vi "Process.vi"(8 "error in":errorcluster, 11 "Logger.Error":refnum<class "Logger.Error.lvclass">) -> (0 "error out":errorcluster, 3 "Logger.Error out":refnum<class "Logger.Error.lvclass">)   [LabVIEW 2019, in "Logger.Error.lvclass"]
doc: "---------------------------------------------------------------\nJKI State Machine Objects™\nhttp://jki.net/state-machine-objects/\nCopyright (C) 2005-2015, JKI <info@jki.net>\nALL RIGHTS RESERVED"
uses:
  Logger.Error.lvclass
  C:/Program Files (x86)/National Instruments/LabVIEW 2019/vi.lib/JKI/JKI SMO/SMO/SMO.lvclass
  C:/Users/patrick/Documents/GitHub/Instrument-Framework/lvsrc/SMOs/Logger/Logger.lvclass
  <vilib>/JKI/JKI SMO/SMO/SMO.lvclass
  <vilib>/JKI/JKI SMO/SMO/SMO.lvclass/SMO.ctl
  Logger.Error.lvclass/Logger.Error.ctl
  <vilib>/JKI/JKI SMO/SMO/Private/ReftoDVR--SMO.vi
  <vilib>/Utility/file.llb/Write Delimited Spreadsheet (string).vi
  <userlib>/LevyLab/Logger/Logger.lvclass
panel:
  out "Status":string
  out "State History":string
  # "error Logger"
  # "For instructions on how to use the JKI State Machine Objects, examples and video tutorials, visit:\nhttp://jki.net/state-machine-objects/\n\nJKI State Machine Objects™\nhttp://jki.net/state-machine-objects/\nCopyright (C) 2005-2015, JKI <info@jki.net>\nALL RIGHTS RESERVED"
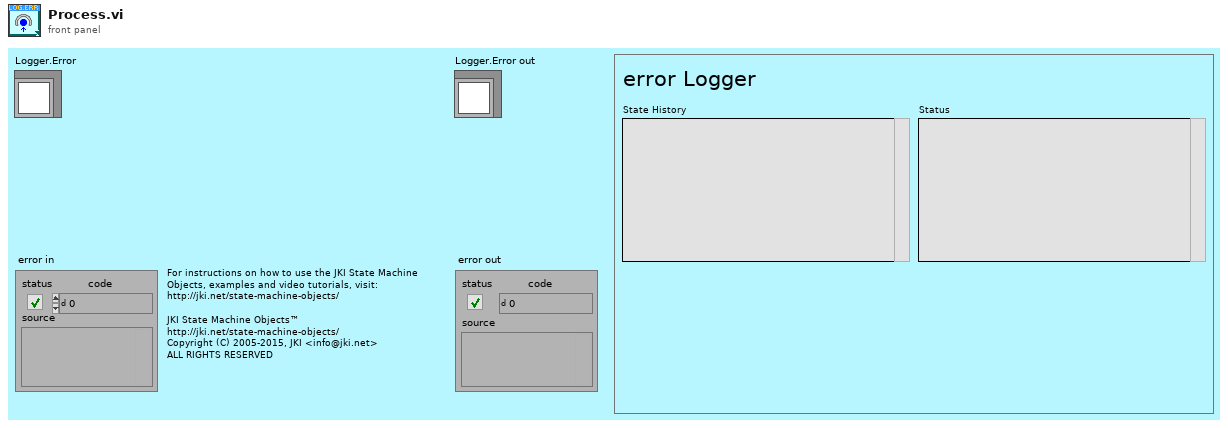
[diagram p1: front panel]
types:
  T1 = enum32{"invalid app kind", "Development System", "Run Time System", "Student Edition", "Embedded LabVIEW", "Evaluation", "Custom"}
  T2 = enum32{"Invalid", "Standard", "Closed", "Hidden", "Minimized", "Maximized"}
  T3 = cluster{"Core":cluster{"Current VI Reference":refnum<vi>, "Close Panel on Exit?":bool, "Last Error":cluster{"error":errorcluster, "previous state":string, "remaining states":string}, "Shutdown?":bool}, "SelfRef":refnum<class "Logger.Error.lvclass">, "path":path, "Debug Mode?":bool, "SMOs":refnum<class "SMO.lvclass">[], "error to log":errorcluster}
  T4 = cluster{"Current VI Reference":refnum<vi>, "Close Panel on Exit?":bool, "Last Error":cluster{"error":errorcluster, "previous state":string, "remaining states":string}, "Shutdown?":bool}
  T5 = typedef "SMO.lvclass/Protected Events.ctl" = cluster{"StopProcesses":refnum<user-event>, "AbortProcesses":refnum<user-event>, "Config Changed":refnum<user-event>, "Dependency":refnum<user-event>}
  T6 = typedef "SMO.lvclass/Public Events.ctl" = cluster{"Error":refnum<user-event>, "State":refnum<user-event>, "Reserve State":refnum<user-event>}
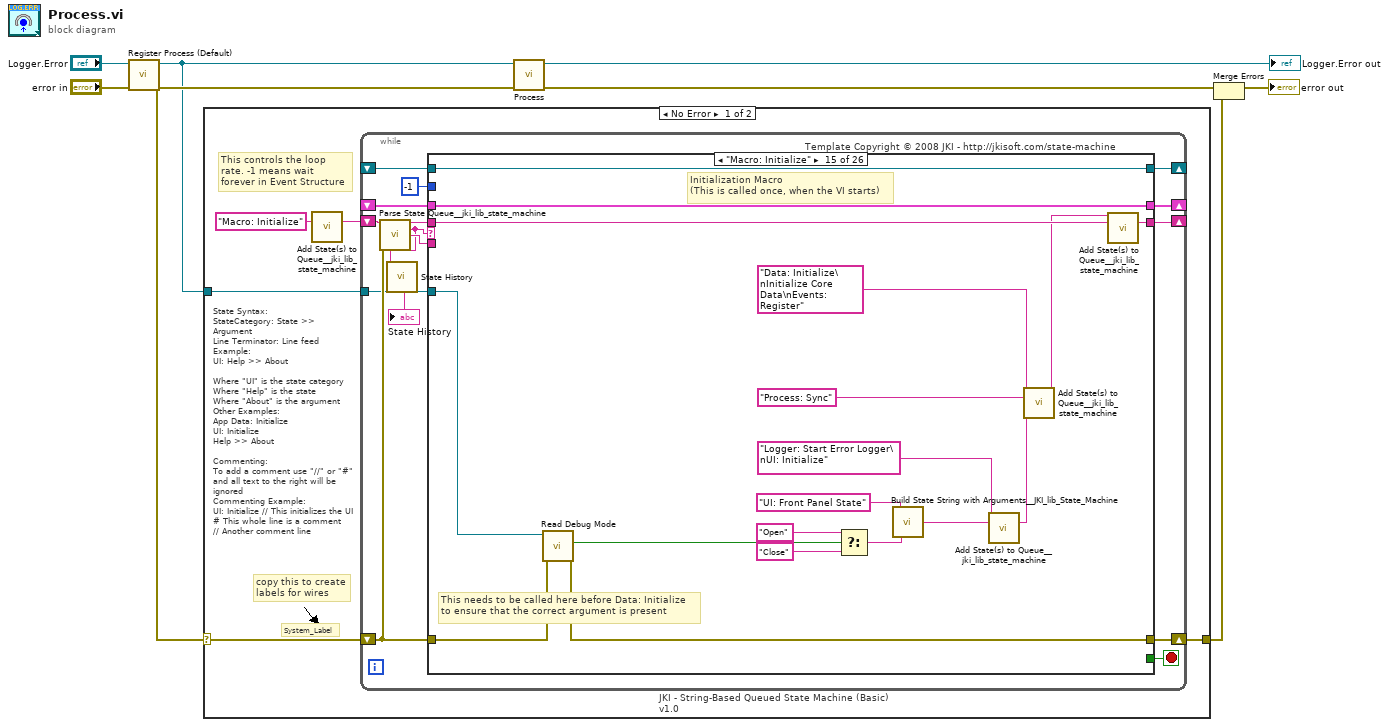
[diagram p0: block diagram]
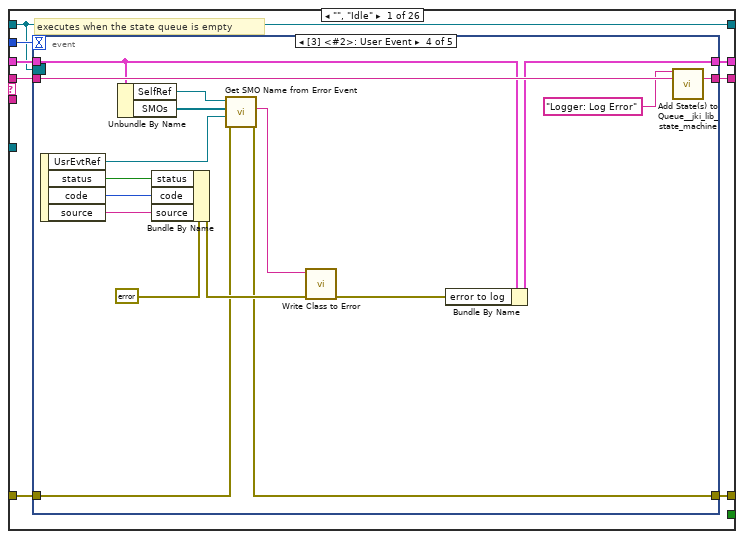
[diagram p2: hidden frame]
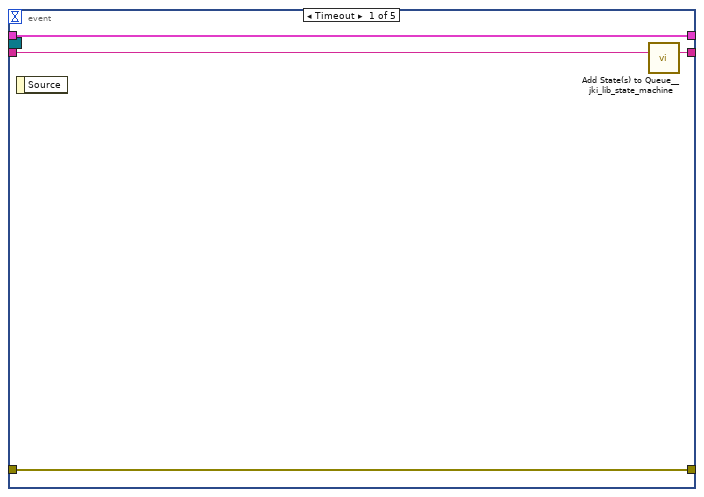
[diagram p3: hidden frame]
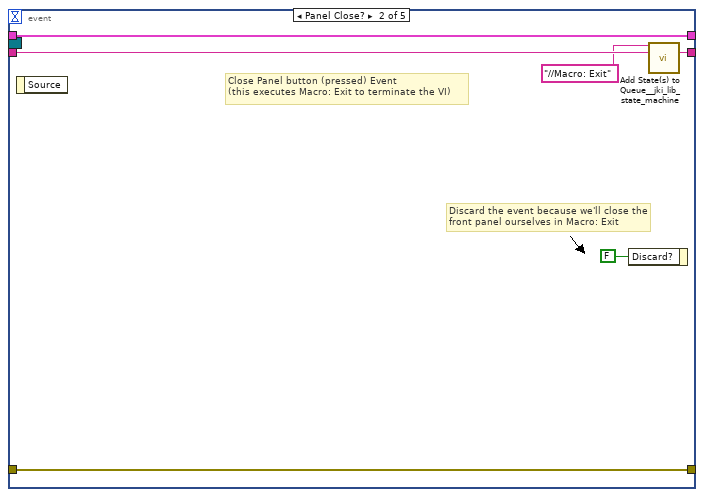
[diagram p4: hidden frame]
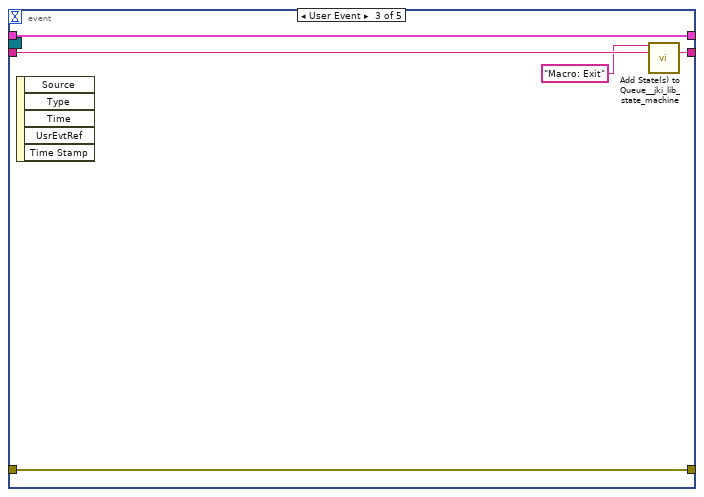
[diagram p5: hidden frame]
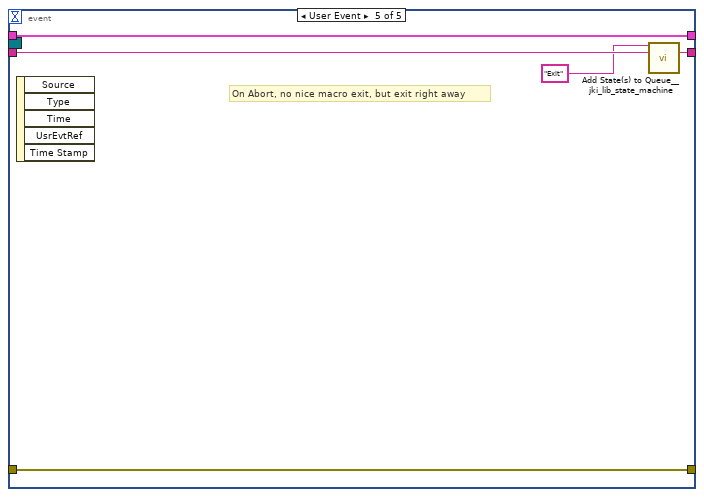
[diagram p6: hidden frame]
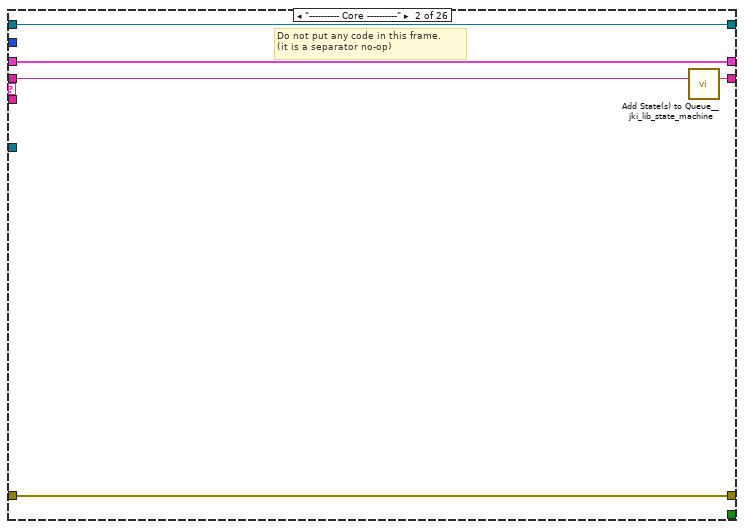
[diagram p7: hidden frame]
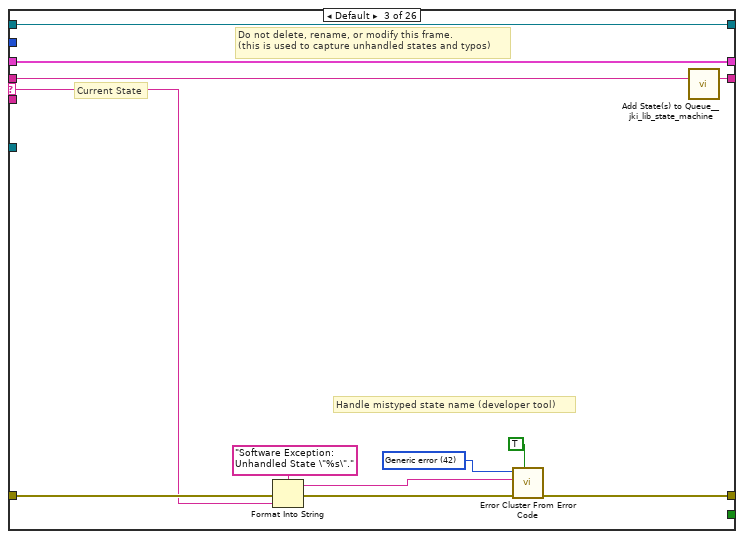
[diagram p8: hidden frame]
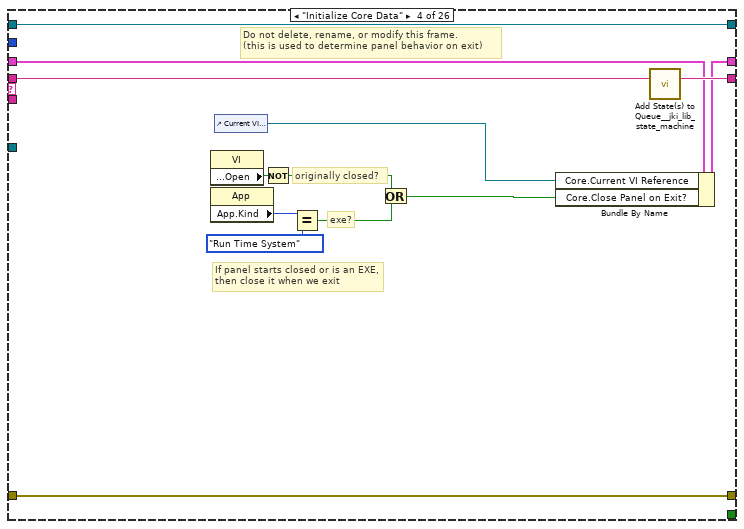
[diagram p9: hidden frame]
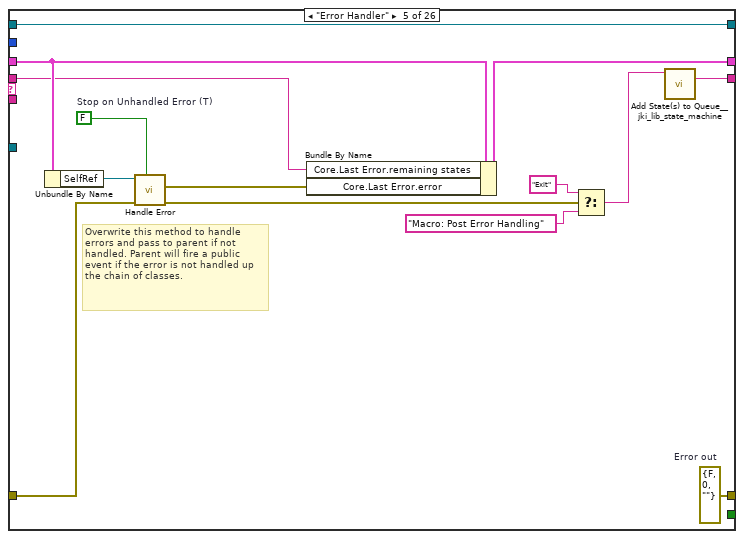
[diagram p10: hidden frame]
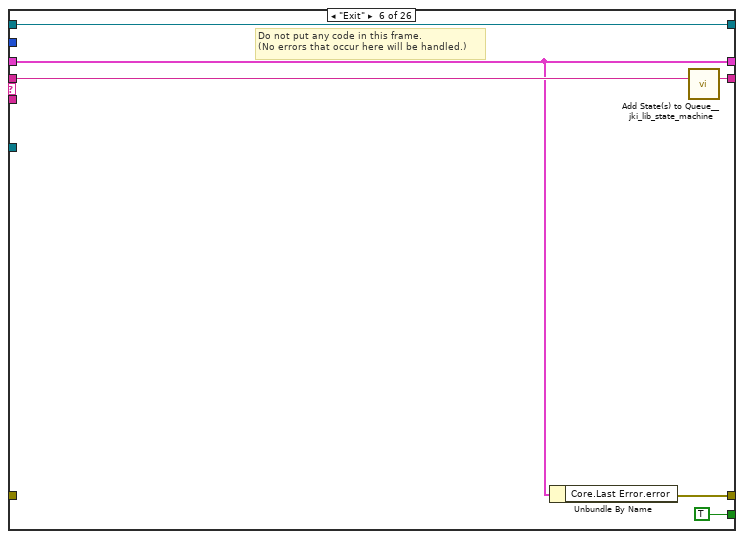
[diagram p11: hidden frame]
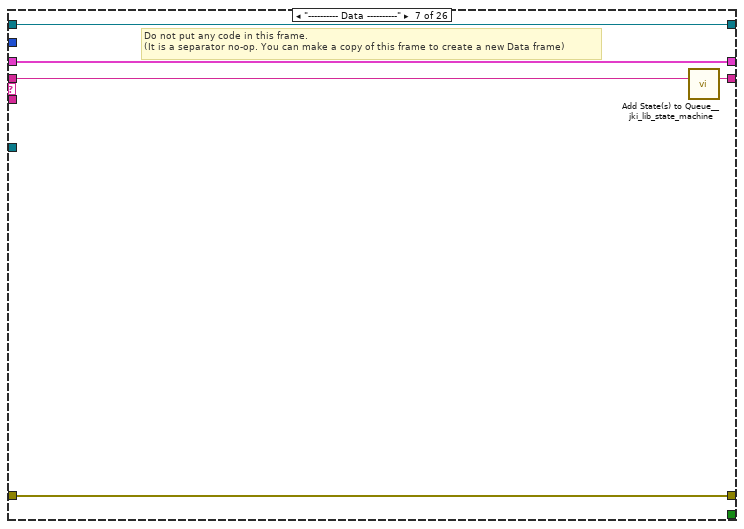
[diagram p12: hidden frame]
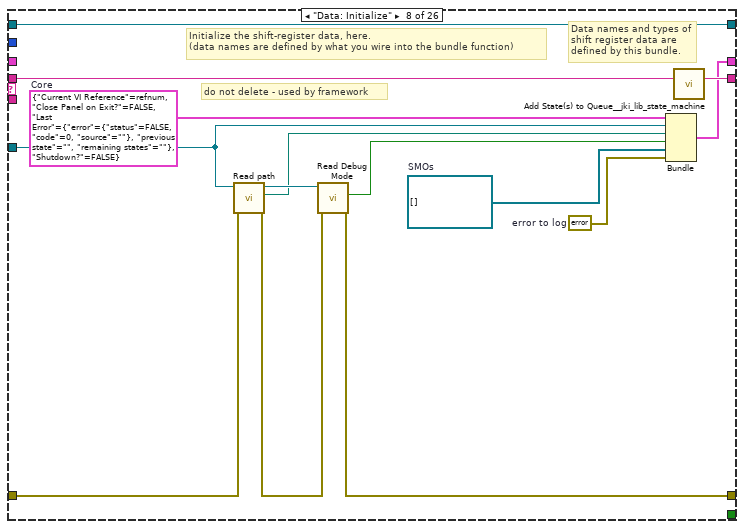
[diagram p13: hidden frame]
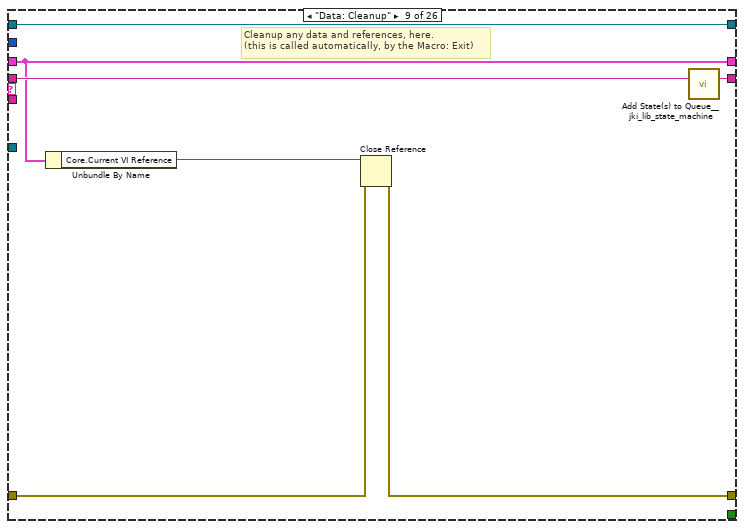
[diagram p14: hidden frame]
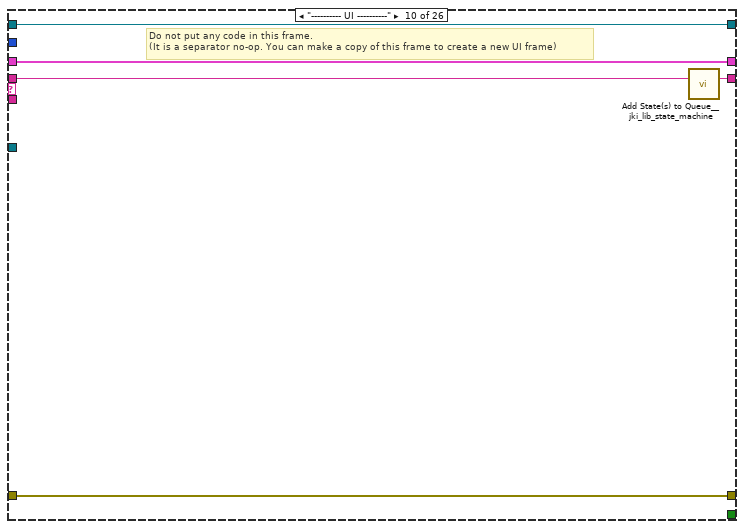
[diagram p15: hidden frame]
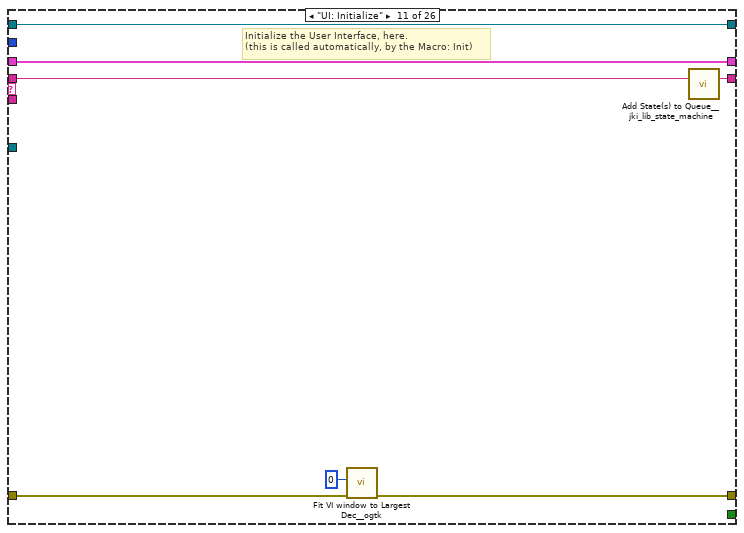
[diagram p16: hidden frame]
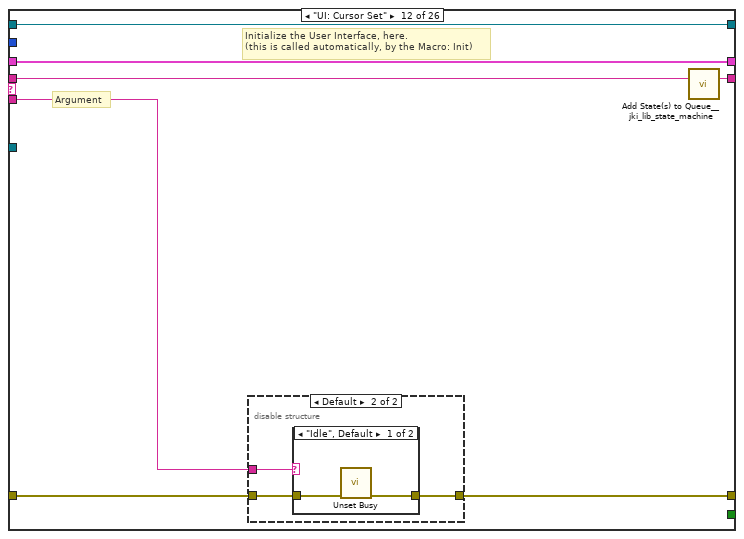
[diagram p17: hidden frame]
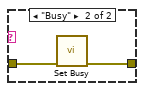
[diagram p19: hidden frame]
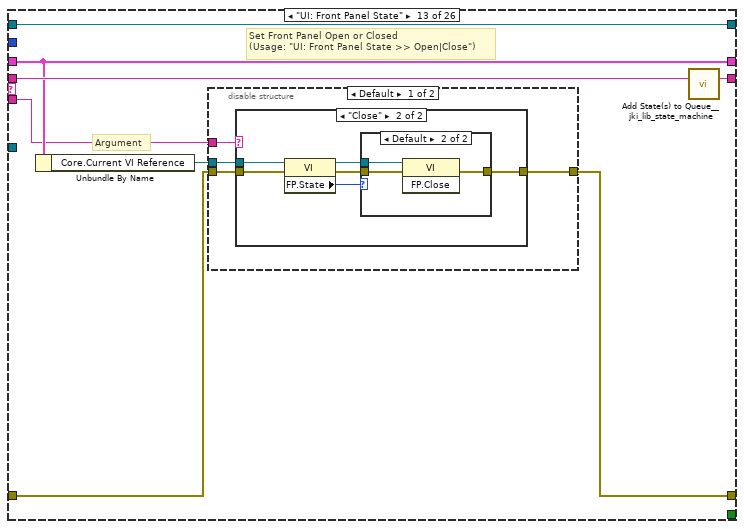
[diagram p20: hidden frame]
diagram:
  n1 = call <vilib>:"Register Process (Default).vi"("error in (no error)"="error in", "SMO"="Logger.Error") -> ("error out"=w5:errorcluster, "SelfRef"=w4:refnum<class "Logger.Error.lvclass">)  [unwired: 8 in]
  n2 = case shown="No Error" w5 {
    selector: w5 -> [w10 w358]
    tunnel: w4 -> [w11 _]
    tunnel: [w9 w358] -> w1
    frame No Error {
      # "State Syntax:\nStateCategory: State >> Argument\nLine Terminator: Line feed\nExample:\nUI: Help >> About\n\nWhere \"UI\" is the state category\nWhere \"Help\" is the state\nWhere \"About\" is the argument\nOther Examples:\nApp Data: Initialize\nUI: Initialize\nHelp >> About\n\nCommenting:\nTo add a comment use \"//\" or \"#\" and all text to the right will be ignored\nCommenting Example:\nUI: Initialize // This initializes the UI\n# This whole line is a comment\n// Another comment line"
      # "copy this to create labels for wires"
      # "This controls the loop rate. -1 means wait forever in Event Structure"
      # "System_Label"
      n3 = call <vilib>:"Add State(s) to Queue__jki_lib_state_machine.vi"("State(s) in (\"\")"="Macro: Initialize") -> ("States Out"=w13:string)  [unwired: 14 in]
      n4 = while "JKI - String-Based Queued State Machine (Basic) v1.0" {
        shift-right: [w22] -> _
        shift-left: _ -> [w14]
        shift-right: [w25] -> w9
        shift-left: w10 -> [w20]
        shift-right: [w24] -> _
        shift-left: w13 -> [w26]
        tunnel: w11 -> [w19]
        shift-right: [w18] -> _
        shift-left: _ -> [w17]
        stop <- w23 stop-if-true
        # "Template Copyright © 2008 JKI - http://jkisoft.com/state-machine"
        n5 = call <vilib>:"Parse State Queue__jki_lib_state_machine.vi"("State Queue"=w26, "Error In (no error)"=w20) -> ("Remaining States"=w28:string, "Current State"=w15:string, "Arguments"=w27:string)  [unwired: 11 in]
        n6 = call <userlib>:"State History.vi"("Current State"=w15) -> ("History"=→"State History":string)  [unwired: 10 in]
        n7 = case shown="\"Macro: Initialize\"" w15 {
          selector: w15 -> [_ _ w80 _ _ _ _ _ _ _ _ _ _ _ _ _ _ _ _ _ _ _ _ _ _ _]
          tunnel: w28 -> [w36 w78 w84 w103 w106 w123 w128 w142 w149 w154 w161 w168 w184 w216 w234 w246 w270 w275 w286 w291 w308 w319 w324 w333 w340 w357]
          tunnel: w27 -> [_ _ _ _ _ _ _ _ _ _ _ w162 w178 _ _ _ _ _ _ _ _ _ _ _ _ _]
          tunnel: [w33 w76 w86 w100 w113 w118 w126 w133 w145 w152 w156 w163 w181 w214 w219 w244 w268 w273 w277 w289 w304 w315 w320 w329 w334 w342] -> w25
          tunnel: w20 -> [w32 w76 w85 w100 w114 _ w126 w129 w146 w152 w155 w164 w182 w214 w218 w244 w268 w273 w278 w289 w295 w315 w320 w330 w335 w347]
          tunnel: [w35 w77 w83 w102 w117 w122 w127 w141 w148 w153 w160 w167 w183 w215 w233 w245 w269 w274 w285 w290 w307 w318 w323 w332 w339 w356] -> w24
          tunnel: [_ _ _ _ _ TRUE _ _ _ _ _ _ _ _ _ _ _ _ _ _ _ _ _ _ _ _] -> w23
          tunnel: [w31 w75 w82 w101 w111 w119 w125 w140 w144 w151 w159 w166 w180 w213 w222 w236 w262 w272 w283 w288 w298 w317 w322 w326 w337 w354] -> w22
          tunnel: -1 ("Timeout") -> [w30 _ _ _ _ _ _ _ _ _ _ _ _ _ _ _ _ _ _ _ _ _ _ _ _ _]
          tunnel: w19 -> [_ _ _ _ _ _ _ w130 _ _ _ _ _ _ w220 _ _ _ _ _ _ _ _ _ _ _]
          tunnel: [w29 w74 w79 w91 w116 w120 w124 w139 w143 w150 w158 w165 w177 w212 w232 w243 w263 w271 w284 w287 w306 w316 w321 w331 w338 w355] -> w18
          tunnel: w17 -> [w29 w74 w79 w91 w116 w120 w124 w139 w143 w150 w158 w165 w177 w212 w232 w243 w263 w271 w284 w287 _ w316 w321 w331 w338 w355]
          tunnel: w14 -> [w34 w75 w82 w94 w112 w119 w125 _ w144 w151 w159 w166 w180 w213 w222 w235 w262 w272 w283 w288 w299 w317 w322 w325 w337 w354]
          frame "", "Idle" {
            # "executes when the state queue is empty"
            n8 = event shown="[3] <#2>: User Event" {
              selector: w29 -> [_ _ _ _ _]
              dyn-events: _ -> [_ _ _ _ _]
              timeout: w30 -> [_ _ _ _ _]
              tunnel: w36 -> [w40 w46 w51 w68 w73]
              tunnel: [w39 w45 w50 w67 w72] -> w35
              tunnel: w34 -> [w38 w43 w48 w55 w70]
              tunnel: [w37 w44 w49 w57 w71] -> w33
              tunnel: w32 -> [w37 w44 w49 w58 w71]
              tunnel: [w38 w43 w48 w56 w70] -> w31
              event Timeout {
                n9 = event-data() -> ()  [unwired: 1 in, 1 out]
                n10 = call <vilib>:"Add State(s) to Queue__jki_lib_state_machine.vi"("State(s) in (\"\")"=w40) -> ("States Out"=w39:string)  [unwired: 14 in]
              }
              event Panel Close? {
                # "Discard the event because we'll close the front panel ourselves in Macro: Exit"
                # "Close Panel button (pressed) Event\n(this executes Macro: Exit to terminate the VI)"
                n11 = event-data() -> ()  [unwired: 1 in, 1 out]
                n12 = event-data("Discard?"=FALSE) -> ()  [unwired: 1 in, 1 out]
                n13 = call <vilib>:"Add State(s) to Queue__jki_lib_state_machine.vi"("State(s) in Front (\"\")"="//Macro: Exit", "State(s) in (\"\")"=w46) -> ("States Out"=w45:string)  [unwired: 13 in]
              }
              event User Event {
                n14 = event-data() -> ()  [unwired: 1 in, 5 out]
                n15 = call <vilib>:"Add State(s) to Queue__jki_lib_state_machine.vi"("State(s) in Front (\"\")"="Macro: Exit", "State(s) in (\"\")"=w51) -> ("States Out"=w50:string)  [unwired: 13 in]
              }
              event User Event {
                n16 = event-data() -> ("UsrEvtRef"=w62:refnum<user-event>, "status"=w66:bool, "code"=w65:i32, "source"=w64:string)  [unwired: 1 in]
                n17 = Unbundle By Name(w55) -> ("SelfRef"=w52:refnum<class "Logger.Error.lvclass">, "SMOs"=w63:refnum<class "SMO.lvclass">[])
                n18 = Bundle By Name(cluster=errorcluster {"status"=FALSE, "code"=0, "source"=""} ("error in (no error)"), "status"=w66, "code"=w65, "source"=w64) -> (w60:errorcluster)
                n19 = call "Get SMO Name from Error Event.vi"("error in (no error)"=w58, "Error"=w62, "SMOs"=w63, "Logger.Error"=w52) -> ("error out"=w57:errorcluster, "class:SMO name"=w61:string)  [unwired: 5 in, 1 out]
                n20 = call "Write Class to Error.vi"("Error in"=w60, "Calling Class"=w61) -> ("Error out"=w54:errorcluster)  [unwired: 9 in]
                n21 = Bundle By Name(cluster=w55, "error to log"=w54) -> (w56:T3)
                n22 = call <vilib>:"Add State(s) to Queue__jki_lib_state_machine.vi"("State(s) in Front (\"\")"="Logger: Log Error" ("State(s) in Front (\"\")"), "State(s) in (\"\")"=w68) -> ("States Out"=w67:string)  [unwired: 13 in]
              }
              event User Event {
                # "On Abort, no nice macro exit, but exit right away"
                n23 = event-data() -> ()  [unwired: 1 in, 5 out]
                n24 = call <vilib>:"Add State(s) to Queue__jki_lib_state_machine.vi"("State(s) in Front (\"\")"="Exit", "State(s) in (\"\")"=w73) -> ("States Out"=w72:string)  [unwired: 13 in]
              }
            }
          }
          frame "---------- Core ----------" {
            # "Do not put any code in this frame.\n(it is a separator no-op)"
            n25 = call <vilib>:"Add State(s) to Queue__jki_lib_state_machine.vi"("State(s) in (\"\")"=w78) -> ("States Out"=w77:string)  [unwired: 14 in]
          }
          frame Default {
            w89 = 42 items=["No error", "Argument error", "Memory is full", "Out of zone", "End of file", "File already open", "Generic file I/O error", "File not found", "File permission error", "Disk is full", "Duplicate path", "Too many files open", "System feature not enabled", "Resource file not found", "Cannot add resource", "Resource not found", "Image not found", "Image memory error", "Pen does not exist", "Config type invalid", "Config token not found", "Config parse error", "Config memory error", "Bad external code format", "Bad external code offset", "External code not present", "Null window", "Destroy window error", "Null menu", "Print aborted", "Bad print record", "Print driver error", "Windows error during printing", "Memory error during printing", "Print dialog error", "Generic print error", "Invalid device refnum", "Device not found", "Device parameter error", "Device unit error", "Cannot open device", "Device call aborted", "Generic error", "Cancelled by user", "Object ID too low", "Object ID too high", "Object not in heap", "Unknown heap", "Unknown object (invalid DefProc)", "Unknown object (DefProc not in table)", "Message out of range", "Invalid (null) method", "Unknown message", "Manager call not supported", "Bad address", "Network operation in progress", "Network operation timed out", "Connection is busy", "Network attribute not supported", "Network error", "Address in use", "System out of memory", "Connection aborted", "Connection refused", "Not connected", "Already connected", "Connection closed", "Initialization error (interapplication manager)", "Bad occurrence", "Wait on unbound occurrence handler", "Occurrence queue overflow", "Datalog type conflict", "Unused", "Unrecognized type (interapplication manager)", "Memory corrupt", "Failed to make temporary DLL", "Old CIN version", "Drag socket not found", "Failed to load drop-object", "Failed to register OLE object", "Failed to release OLE object", "Format specifier type mismatch", "Unknown format specifier", "Too few format specifiers", "Too many format specifiers", "Scan failed", "Newer CIN version", "Error converting to variant", "Runtime menu error", "Password tampered", "Variant attribute not found", "Incompatible variant data type", "Event data is not available", "Event Store is not present", "Occurrence is not found", "Event Queue is not created", "Event info is not available", "Refnum passed is NULL", "Error retrieving Class GUID", "Error retrieving CoClass GUID", "Error retrieving TypeLib GUID.", "Bad built application magic bytes.", "Specific driver is different from the specific driver associated with the Logical Name.", "There is no session opened to the class driver.", "Max Error", "MAX - Error with config objects", "MAX - Error loading configuration", "MAX - Group not supported"]
            # "Current State"
            # "Do not delete, rename, or modify this frame.\n(this is used to capture unhandled states and typos)"
            # "Handle mistyped state name (developer tool)"
            n26 = Format Into String(format string="Software Exception: Unhandled State \"%s\"." ("message"), error in=w85, w80) -> (resulting string=w88:string, error out=w87:errorcluster)  [unwired: 1 in]
            n27 = call <vilib>:"Error Cluster From Error Code.vi"("show call chain? (False)"=TRUE, "error in (no error)"=w87, "error message (\"\")"=w88, "error code (0)"=w89) -> ("error out"=w86:errorcluster)  [unwired: 5 in]
            n28 = call <vilib>:"Add State(s) to Queue__jki_lib_state_machine.vi"("State(s) in (\"\")"=w84) -> ("States Out"=w83:string)  [unwired: 14 in]
          }
          frame "Initialize Core Data" {
            # "Do not delete, rename, or modify this frame.\n(this is used to determine panel behavior on exit)"
            # "originally closed?"
            # "exe?"
            # "If panel starts closed or is an EXE, then close it when we exit"
            n29 = property class="VI"() -> ("Front Panel.Open"=w99:bool)  [unwired: 2 in, 2 out]
            n30 = property class="App"() -> ("App.Kind"=w98:T1)  [unwired: 2 in, 2 out]
            n31 = control-ref of="Current VI Reference"() -> (w92:refnum<vi>)
            n32 = Not(x=w99) -> (.not. x?=w96:bool)
            n33 = Equal?(x=w98, y=T1."Run Time System" ("Application:Kind")) -> (x = y?=w95:bool)
            n34 = Or(x=w96, y=w95) -> (x .or. y?=w93:bool)
            n35 = Bundle By Name(cluster=w94, "Core.Current VI Reference"=w92, "Core.Close Panel on Exit?"=w93) -> (w101:T3)
            n36 = call <vilib>:"Add State(s) to Queue__jki_lib_state_machine.vi"("State(s) in (\"\")"=w103) -> ("States Out"=w102:string)  [unwired: 14 in]
          }
          frame "Error Handler" {
            w107 = FALSE  # Stop on Unhandled Error (T)
            w113 = errorcluster {"status"=FALSE, "code"=0, "source"=""}  # Error out
            # "Overwrite this method to handle errors and pass to parent if not handled. Parent will fire a public event if the error is not handled up the chain of classes."
            n37 = Unbundle By Name(w112) -> ("SelfRef"=w115:refnum<class "Logger.Error.lvclass">)
            n38 = call-dynamic "Handle Error.vi"("Stop on Unhandled Error (T)"=w107, "error in"=w114, "SMO"=w115) -> ("handling error"=w108:errorcluster, "Unhandled error"=w104:errorcluster)  [unwired: 6 in, 1 out]
            n39 = Bundle By Name(cluster=w112, "Core.Last Error.remaining states"=w106, "Core.Last Error.error"=w104) -> (w111:T3)
            n40 = Select(t="Exit", s=w108, f="Macro: Post Error Handling") -> (s? t:f=w110:string)
            n41 = call <vilib>:"Add State(s) to Queue__jki_lib_state_machine.vi"("State(s) in Front (\"\")"=w110) -> ("States Out"=w117:string)  [unwired: 14 in]
          }
          frame "Exit" {
            # "Do not put any code in this frame.\n(No errors that occur here will be handled.)"
            n42 = Unbundle By Name(w119) -> ("Core.Last Error.error"=w118:errorcluster)
            n43 = call <vilib>:"Add State(s) to Queue__jki_lib_state_machine.vi"("State(s) in (\"\")"=w123) -> ("States Out"=w122:string)  [unwired: 14 in]
          }
          frame "---------- Data ----------" {
            # "Do not put any code in this frame.\n(It is a separator no-op. You can make a copy of this frame to create a new Data frame)"
            n44 = call <vilib>:"Add State(s) to Queue__jki_lib_state_machine.vi"("State(s) in (\"\")"=w128) -> ("States Out"=w127:string)  [unwired: 14 in]
          }
          frame "Data: Initialize" {
            w131 = errorcluster {"status"=FALSE, "code"=0, "source"=""}  # error to log
            w132 = refnum<class "SMO.lvclass">[] []  # SMOs
            w138 = T4 {"Current VI Reference"=refnum, "Close Panel on Exit?"=FALSE, "Last Error"={"error"={"status"=FALSE, "code"=0, "source"=""}, "previous state"="", "remaining states"=""}, "Shutdown?"=FALSE}  # Core
            # "do not delete - used by framework"
            # "Data names and types of shift register data are defined by this bundle."
            # "Initialize the shift-register data, here.\n(data names are defined by what you wire into the bundle function)"
            n45 = call-dynamic "Read path.vi"("error in (no error)"=w129, "Logger in"=w130) -> ("error out"=w135:errorcluster, "path"=w134:path, "Logger out"=w137:refnum<class "Logger.Error.lvclass">)  [unwired: 7 in]
            n46 = call <userlib>:"Read Debug Mode.vi"("error in (no error)"=w135, "Logger in"=w137) -> ("error out"=w133:errorcluster, "Debug Mode?"=w136:bool)  [unwired: 7 in, 1 out]
            n47 = Bundle("Core"=w138, "SelfRef"=w130, "path"=w134, "Debug Mode?"=w136, "SMOs"=w132, "error to log"=w131) -> (w140:T3)  [unwired: 1 in]
            n48 = call <vilib>:"Add State(s) to Queue__jki_lib_state_machine.vi"("State(s) in (\"\")"=w142) -> ("States Out"=w141:string)  [unwired: 14 in]
          }
          frame "Data: Cleanup" {
            # "Cleanup any data and references, here.\n(this is called automatically, by the Macro: Exit)"
            n49 = Unbundle By Name(w144) -> ("Core.Current VI Reference"=w147:refnum<vi>)
            n50 = Close Reference(reference=w147, error in (no error)=w146) -> (error out=w145:errorcluster)
            n51 = call <vilib>:"Add State(s) to Queue__jki_lib_state_machine.vi"("State(s) in (\"\")"=w149) -> ("States Out"=w148:string)  [unwired: 14 in]
          }
          frame "---------- UI ----------" {
            # "Do not put any code in this frame.\n(It is a separator no-op. You can make a copy of this frame to create a new UI frame)"
            n52 = call <vilib>:"Add State(s) to Queue__jki_lib_state_machine.vi"("State(s) in (\"\")"=w154) -> ("States Out"=w153:string)  [unwired: 14 in]
          }
          frame "UI: Initialize" {
            # "Initialize the User Interface, here.\n(this is called automatically, by the Macro: Init)"
            n53 = call <userlib>:"Fit VI window to Largest Dec__ogtk.vi"("error in (no error)"=w155, "border spacing (2 px)"=0) -> ("error out"=w156:errorcluster)  [unwired: 4 in, 1 out]
            n54 = call <vilib>:"Add State(s) to Queue__jki_lib_state_machine.vi"("State(s) in (\"\")"=w161) -> ("States Out"=w160:string)  [unwired: 14 in]
          }
          frame "UI: Cursor Set" {
            # "Argument"
            # "Initialize the User Interface, here.\n(this is called automatically, by the Macro: Init)"
            n55 = disable-structure shown="Default" {
              disable-tunnel: w164 -> [w169 w172]
              disable-tunnel: [w169 w171] -> w163
              disable-tunnel: w162 -> [_ w170]
              frame condition #0 {
              }
              frame condition #1 (active) {
                n56 = case shown="\"Idle\", Default" w170 {
                  tunnel: w172 -> [w174 w176]
                  tunnel: [w173 w175] -> w171
                  frame "Idle", Default {
                    n57 = call <vilib>:"Unset Busy.vi"("error in (no error)"=w174) -> ("error out"=w173:errorcluster)  [unwired: 10 in]
                  }
                  frame "Busy" {
                    n58 = call <vilib>:"Set Busy.vi"("error in (no error)"=w176) -> ("error out"=w175:errorcluster)  [unwired: 9 in, 1 out]
                  }
                }
              }
            }
            n59 = call <vilib>:"Add State(s) to Queue__jki_lib_state_machine.vi"("State(s) in (\"\")"=w168) -> ("States Out"=w167:string)  [unwired: 14 in]
          }
          frame "UI: Front Panel State" {
            # "Argument"
            # "Set Front Panel Open or Closed\n(Usage: \"UI: Front Panel State >> Open|Close\")"
            n60 = Unbundle By Name(w180) -> ("Core.Current VI Reference"=w179:refnum<vi>)
            n61 = disable-structure shown="Default" {
              disable-tunnel: w182 -> [w188 w211]
              disable-tunnel: [w187 w211] -> w181
              disable-tunnel: w179 -> [w186 _]
              disable-tunnel: w178 -> [w185 _]
              frame condition #0 (active) {
                n62 = case shown="\"Close\"" w185 {
                  tunnel: w188 -> [w192 w205]
                  tunnel: [w194 w206] -> w187
                  tunnel: w186 -> [w193 w203]
                  frame "Open", Default {
                    n63 = property class="VI"(reference=w193, error in=w192) -> (reference out=w190:refnum<vi>, error out=w191:errorcluster, "FP.State"=w189:T2)
                    n64 = case shown="\"Closed\"" w189 {
                      tunnel: [w197 w200] -> w194
                      tunnel: w191 -> [w196 w200]
                      tunnel: w190 -> [w195 _]
                      frame "Closed" {
                        n65 = invoke class="VI" method="FP.Open"(reference=w195, error in=w196, "Activate"=TRUE, "State"=T2."Standard") -> (error out=w197:errorcluster)  [unwired: 1 in, 4 out]
                      }
                      frame Default {
                      }
                    }
                  }
                  frame "Close" {
                    n66 = property class="VI"(reference=w203, error in=w205) -> (reference out=w202:refnum<vi>, error out=w204:errorcluster, "FP.State"=w201:T2)
                    n67 = case shown="Default" w201 {
                      tunnel: [w207 w210] -> w206
                      tunnel: w204 -> [w207 w209]
                      tunnel: w202 -> [_ w208]
                      frame "Invalid", "Closed" {
                      }
                      frame Default {
                        n68 = invoke class="VI" method="FP.Close"(reference=w208, error in=w209) -> (error out=w210:errorcluster)  [unwired: 1 in, 2 out]
                      }
                    }
                  }
                }
              }
              frame condition #1 {
              }
            }
            n69 = call <vilib>:"Add State(s) to Queue__jki_lib_state_machine.vi"("State(s) in (\"\")"=w184) -> ("States Out"=w183:string)  [unwired: 14 in]
          }
          frame "---------- Macro ----------" {
            # "Do not put any code in this frame.\n(It is a separator no-op. You can make a copy of this frame to create a new Macro frame)"
            n70 = call <vilib>:"Add State(s) to Queue__jki_lib_state_machine.vi"("State(s) in (\"\")"=w216) -> ("States Out"=w215:string)  [unwired: 14 in]
          }
          frame "Macro: Initialize" {
            # "This needs to be called here before Data: Initialize\nto ensure that the correct argument is present"
            # "Initialization Macro\n(This is called once, when the VI starts)"
            n71 = call <userlib>:"Read Debug Mode.vi"("error in (no error)"=w218, "Logger in"=w220) -> ("error out"=w219:errorcluster, "Debug Mode?"=w217:bool)  [unwired: 7 in, 1 out]
            n72 = Select(t="Open", s=w217, f="Close") -> (s? t:f=w226:string)
            n73 = call <vilib>:"Build State String with Arguments__JKI_lib_State_Machine.vi"("Arguments (\"\")"=w226, "State"="UI: Front Panel State") -> ("State with Arguments"=w223:string)  [unwired: 4 in]
            n74 = call <vilib>:"Add State(s) to Queue__jki_lib_state_machine.vi"("State(s) in Front (\"\")"="Logger: Start Error Logger\nUI: Initialize", "State(s) in (\"\")"=w223) -> ("States Out"=w221:string)  [unwired: 13 in]
            n75 = call <vilib>:"Add State(s) to Queue__jki_lib_state_machine.vi"("State(s) in Front (\"\")"="Data: Initialize\nInitialize Core Data\nEvents: Register", "State(s) in (\"\")"="Process: Sync", "State(s) at Back (\"\")"=w221) -> ("States Out"=w230:string)  [unwired: 12 in]
            n76 = call <vilib>:"Add State(s) to Queue__jki_lib_state_machine.vi"("State(s) in Front (\"\")"=w230, "State(s) in (\"\")"=w234) -> ("States Out"=w233:string)  [unwired: 13 in]
          }
          frame "Macro: Post Error Handling" {
            # "Clear Last Error?"
            n77 = Unbundle By Name(w235) -> ("Core.Last Error.remaining states"=w238:string, "Core.Shutdown?"=w239:bool)
            n78 = Unbundle By Name(w235) -> ("Core.Last Error.error"=w242:errorcluster)
            n79 = case shown="False" FALSE {
              tunnel: w242 -> [w250 _]
              tunnel: [w250 _] -> w241
              frame False {
              }
              frame True {
              }
            }
            n80 = case shown="False" w239 {
              tunnel: w238 -> [w247 w249]
              tunnel: [w247 w248] -> w237
              frame False {
                # "These are the remaining states (at the moment the error occured). States can be altered according to business logic."
                # "NOT SHUTTING DOWN"
              }
              frame True {
                # "Developer can decide to alter the states but should be aware that during the shutdown process, there are certain states that must be run for the SMO to properly shut itself (and this process) down. As such, one can add states to perform additional clean-ups, but should append the remaining state to be executed."
                # "SHUTTING DOWN"
                n81 = call <vilib>:"Add State(s) to Queue__jki_lib_state_machine.vi"("State(s) in (\"\")"=w249) -> ("States Out"=w248:string)  [unwired: 14 in]
              }
            }
            n82 = Bundle By Name(cluster=w235, "Core.Last Error.error"=w241) -> (w236:T3)
            n83 = call <vilib>:"Add State(s) to Queue__jki_lib_state_machine.vi"("State(s) in Front (\"\")"=w237, "State(s) in (\"\")"=w246) -> ("States Out"=w245:string)  [unwired: 13 in]
          }
          frame "Macro: Exit" {
            # "Exit Macro\n(This is called once, when the VI exits)"
            n84 = Unbundle By Name(w262) -> ("Debug Mode?"=w251:bool, "Core.Close Panel on Exit?"=w267:bool)
            n85 = Select(t="Open", s=w251, f="Close") -> (s? t:f=w254:string)
            n86 = call <vilib>:"Build State String with Arguments__JKI_lib_State_Machine.vi"("Arguments (\"\")"=w254, "State"="UI: Front Panel State") -> ("State with Arguments"=w252:string)  [unwired: 4 in]
            n87 = Select(t=w252, s=w267, f="") -> (s? t:f=w265:string)
            n88 = call <vilib>:"Add State(s) to Queue__jki_lib_state_machine.vi"("State(s) in Front (\"\")"="Logger: Stop Error Logger\nData: Cleanup\nEvents: Unregister", "State(s) in (\"\")"="Process: Sync", "State(s) at Back (\"\")"="Exit") -> ("States Out"=w259:string)  [unwired: 12 in]
            n89 = call <vilib>:"Add State(s) to Queue__jki_lib_state_machine.vi"("State(s) in Front (\"\")"="" ("State(s) in Front (\"\")"), "State(s) in (\"\")"=w265, "State(s) at Back (\"\")"=w259) -> ("States Out"=w264:string)  [unwired: 12 in]
            n90 = call <vilib>:"Add State(s) to Queue__jki_lib_state_machine.vi"("State(s) in Front (\"\")"=w264, "State(s) in (\"\")"=w270) -> ("States Out"=w269:string)  [unwired: 13 in]
          }
          frame "---------- Process ----------" {
            # "Template Separator\n(You can make a copy of, or modify, this frame)"
            n91 = call <vilib>:"Add State(s) to Queue__jki_lib_state_machine.vi"("State(s) in (\"\")"=w275) -> ("States Out"=w274:string)  [unwired: 14 in]
          }
          frame "Process: Sync" {
            n92 = Unbundle By Name(w283) -> ("SelfRef"=w279:refnum<class "Logger.Error.lvclass">)
            n93 = call <vilib>:"WaitOnProcessSync.vi"("error in (no error)"=w278, "SMO"=w279) -> ("error out"=w277:errorcluster, "Don't run?"=w282:bool)  [unwired: 7 in, 1 out]
            n94 = Select(t="Data: Cleanup\nEvents: Unregister\nExit", s=w282, f="") -> (s? t:f=w276:string)
            n95 = call <vilib>:"Add State(s) to Queue__jki_lib_state_machine.vi"("State(s) in Front (\"\")"=w276, "State(s) in (\"\")"=w286) -> ("States Out"=w285:string)  [unwired: 13 in]
          }
          frame "---------- Events ----------" {
            # "Template Separator\n(You can make a copy of, or modify, this frame)"
            n96 = call <vilib>:"Add State(s) to Queue__jki_lib_state_machine.vi"("State(s) in (\"\")"=w291) -> ("States Out"=w290:string)  [unwired: 14 in]
          }
          frame "Events: Register" {
            n97 = Unbundle By Name(w299) -> ("SelfRef"=w305:refnum<class "Logger.Error.lvclass">)
            n98 = call <vilib>:"GetProtectedEvents.vi"("SMO"=w305) -> ("error out"=w303:errorcluster, "SMO Protected Events"=w302:T5, "SMO out"=w301:refnum<class "Logger.Error.lvclass">)  [unwired: 8 in]
            n99 = Unbundle By Name(w301) -> ("SMOs"=w293:refnum<class "SMO.lvclass">[])
            n100 = Build Array (concatenate)(w293, w301) -> (w300:refnum<class "SMO.lvclass">[])
            n101 = for {
              tunnel: w300 -> [w312] mode=indexing
              tunnel: [w311] -> w297 mode=indexing
              tunnel: [w309] -> w296 mode=indexing
              tunnel: [w310] -> w292 mode=indexing
              n102 = call <vilib>:"GetPublicEvents.vi"("SMO"=w312) -> ("error out"=w310:errorcluster, "Public Events"=w313:T6, "SMO out"=w309:refnum<class "SMO.lvclass">)  [unwired: 8 in]
              n103 = Unbundle By Name(w313) -> ("Error"=w311:refnum<user-event>)
            }
            n104 = register-events(w302, w297) -> (reference out=w306:refnum<event-registration>, error out=w294:errorcluster)  [unwired: 2 in]
            n105 = Bundle By Name(cluster=w299, "SMOs"=w296) -> (w298:T3)
            n106 = Merge Errors(w294, w292, w303, w295) -> (w304:errorcluster)
            n107 = call <vilib>:"Add State(s) to Queue__jki_lib_state_machine.vi"("State(s) in (\"\")"=w308) -> ("States Out"=w307:string)  [unwired: 14 in]
          }
          frame "Events: Unregister" {
            n108 = Unregister For Events(event registration refnum=w316, error in=w315) -> (error out=w314:errorcluster)
            n109 = call <vilib>:"Clear Errors.vi"("error in (no error)"=w314) -> ()  [unwired: 5 in, 2 out]
            n110 = call <vilib>:"Add State(s) to Queue__jki_lib_state_machine.vi"("State(s) in (\"\")"=w319) -> ("States Out"=w318:string)  [unwired: 14 in]
          }
          frame "---------- Logger ----------" {
            n111 = call <vilib>:"Add State(s) to Queue__jki_lib_state_machine.vi"("State(s) in (\"\")"=w324) -> ("States Out"=w323:string)  [unwired: 14 in]
          }
          frame "Logger: Start Error Logger" {
            # "will these work with other SMOs?"
            n112 = Unbundle By Name(w325) -> ("SelfRef"=w328:refnum<class "Logger.Error.lvclass">)
            n113 = call-dynamic "Create Logger.vi"("error in (no error)"=w330, "Logger.Error in"=w328) -> ("error out"=w329:errorcluster, "Logger.Error out"=w327:refnum<class "Logger.Error.lvclass">)  [unwired: 8 in]
            n114 = Bundle By Name(cluster=w325, "SelfRef"=w327) -> (w326:T3)
            n115 = call <vilib>:"Add State(s) to Queue__jki_lib_state_machine.vi"("State(s) in (\"\")"=w333) -> ("States Out"=w332:string)  [unwired: 14 in]
          }
          frame "Logger: Stop Error Logger" {
            n116 = Unbundle By Name(w337) -> ("SelfRef"=w336:refnum<class "Logger.Error.lvclass">)
            n117 = call-dynamic "Destroy Logger.vi"("error in (no error)"=w335, "Logger.Error in"=w336) -> ("error out"=w334:errorcluster)  [unwired: 8 in, 1 out]
            n118 = call <vilib>:"Add State(s) to Queue__jki_lib_state_machine.vi"("State(s) in (\"\")"=w340) -> ("States Out"=w339:string)  [unwired: 14 in]
          }
          frame "Logger: Log Error" {
            n119 = Unbundle By Name(w354) -> ("SelfRef"=w350:refnum<class "Logger.Error.lvclass">, "error to log"=w352:errorcluster)
            n120 = call-dynamic "Read path.vi"("error in (no error)"=w347, "Logger in"=w350) -> ("error out"=w348:errorcluster, "path"=w349:path)  [unwired: 7 in, 1 out]
            n121 = call "Error Cluster to Array.vi"("error in (no error)"=w352) -> ("Error Array"=w351:string[])  [unwired: 10 in]
            n122 = call-poly <vilib>:"Write Delimited Spreadsheet.vi"("file path (dialog if empty)"=w349, "1D data"=w351, "append to file? (new file:F)"=TRUE, "error in (no error)"=w348) -> ("error out"=w343:errorcluster)  [unwired: 10 in, 1 out]
            n123 = Get Date/Time In Seconds() -> (seconds since 1Jan1904=w345:timestamp)
            n124 = Format Into String(error in=w343, "Error Logged", w345) -> (resulting string=w344:string, error out=w342:errorcluster)  [unwired: 2 in]
            n125 = call <userlib>:"State History.vi"("Current State"=w344) -> ("History"=→"Status":string)  [unwired: 10 in]
            n126 = call <vilib>:"Add State(s) to Queue__jki_lib_state_machine.vi"("State(s) in (\"\")"=w357) -> ("States Out"=w356:string)  [unwired: 14 in]
          }
        }
      }
    }
    frame Error {
    }
  }
  n127 = call-parent "Process.vi"("error in"=w5, "SMO"=w4) -> ("error out"=w2:errorcluster, "SMO out"=→"Logger.Error out":refnum<class "Logger.Error.lvclass">)  [unwired: 8 in]
  n128 = Merge Errors(w2, w1) -> (→"error out":errorcluster)
